vi "Tree Data Types and XML Example.vi"(0 "Show IDs (True)":bool, 1 "Tree":string(tree)) -> (12 "XML String":string)   [LabVIEW 2016, in "Tree Manager.lvclass"]
uses:
  Tree Manager.lvclass
  Data Types/String/String.lvclass/String.ctl
  Data Types/Bool/Bool.lvclass/Bool.ctl
  Data Types/Float/Float.lvclass/Float.ctl
  Data Types/Int/Integer.lvclass/Integer.ctl
  Data Types/Path/Path.lvclass/Path.ctl
  Data Types/Float/To Float Tree Data.vi
  Data Types/Bool/To Bool Tree Data.vi
  Data Types/Path/To Path Tree Data.vi
  Data Types/Int/To Integer Tree Data.vi
  Data Types/String/To String Tree Data.vi
  Data Types/Bool/Bool.lvclass
  C:/Users/plkruczp/Google Drive/MyCode/Modules/Tree/Tree Data/Tree Data.lvclass
  Data Types/Float/Float.lvclass
  Data Types/Int/Integer.lvclass
  Data Types/Path/Path.lvclass
  Data Types/String/String.lvclass
  API/List Roots.vi
  API/Set Attribute Tree Data.vi
  Tree Data/Tree Data.lvclass
  Data Types/Int/From Integer Tree Data.vi
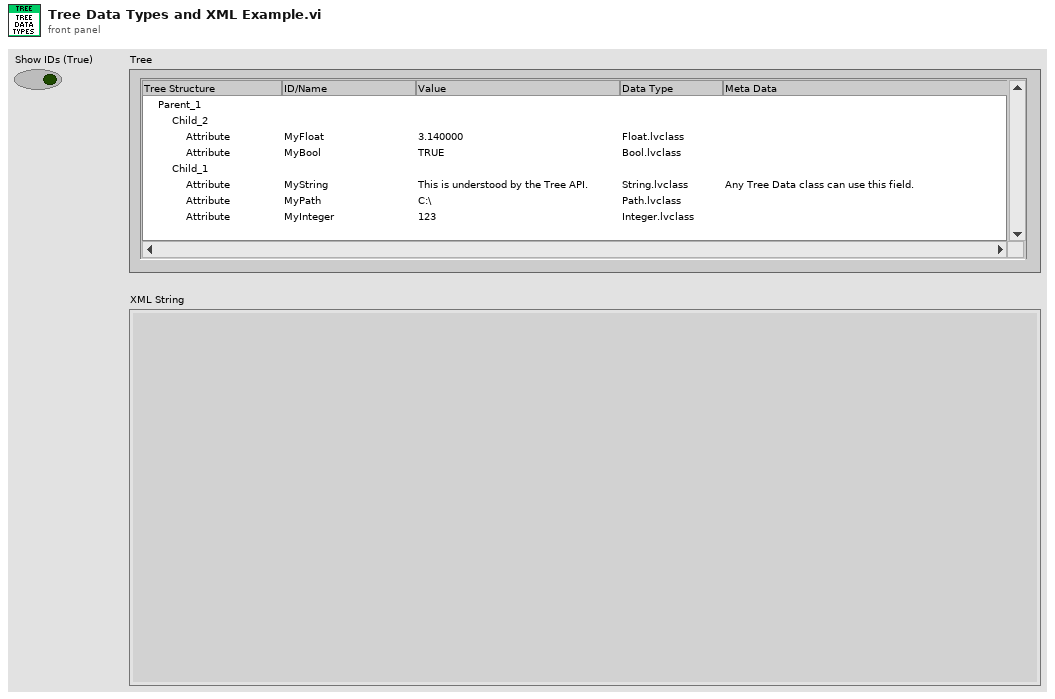
[diagram p1: front panel]
types:
  T1 = typedef "Tree Manager.lvclass/Session Handle.ctl" = refnum<data-value>
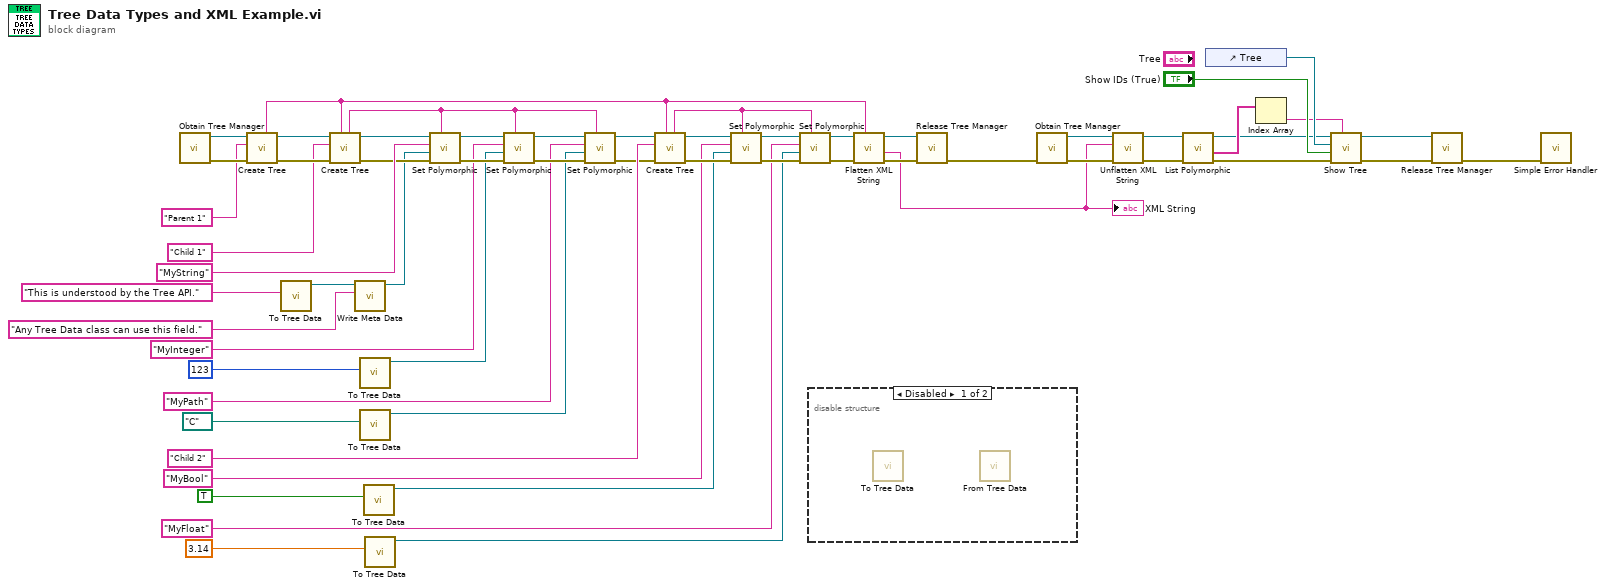
[diagram p0: block diagram]
diagram:
  n1 = call "Obtain Tree Manager.vi"() -> ("Error Out"=w57:errorcluster, "Tree Manager"=w58:T1)  [unwired: 10 in]
  n2 = call "Create Tree.vi"("Error In"=w57, "Name"="Parent 1", "Tree Manager"=w58) -> ("Error Out"=w55:errorcluster, "Tree Manager"=w56:T1, "Unique ID"=w13:string)  [unwired: 6 in]
  n3 = call-poly "To Tree Data.vi"("String"="This is understood by the Tree API.") -> ("String Tree Data"=w22:refnum<class "String.lvclass">)  [unwired: 10 in]
  n4 = call "Create Tree.vi"("Parent ID (empty)"=w13, "Error In"=w55, "Name"="Child 1", "Tree Manager"=w56) -> ("Error Out"=w45:errorcluster, "Tree Manager"=w47:T1, "Unique ID"=w21:string)  [unwired: 5 in]
  n5 = call "Write Meta Data.vi"("Meta Data"="Any Tree Data class can use this field.", "Tree Data In"=w22) -> ("Tree Data Out"=w44:refnum<class "String.lvclass">)  [unwired: 9 in]
  n6 = call-poly "To Tree Data.vi"("Integer"=i64 123) -> ("Integer Tree Data"=w24:refnum<class "Integer.lvclass">)  [unwired: 10 in]
  n7 = call-poly "To Tree Data.vi"("Path"=path "C:/") -> ("Path Tree Data"=w26:refnum<class "Path.lvclass">)  [unwired: 10 in]
  n8 = call-poly "To Tree Data.vi"("Boolean"=TRUE) -> ("Bool Tree Data"=w28:refnum<class "Bool.lvclass">)  [unwired: 10 in]
  n9 = call-poly "To Tree Data.vi"("Float"=3.14) -> ("Float Tree Data"=w30:refnum<class "Float.lvclass">)  [unwired: 10 in]
  n10 = call-poly "Set Polymorphic.vi"("Tree ID"=w21, "Error In"=w45, "Attribute Value"=w44, "Attribute Name"="MyString" ("Name"), "Tree Manager"=w47) -> ("Error Out"=w38:errorcluster, "Tree Manager"=w39:T1)  [unwired: 4 in, 1 out]
  n11 = call-poly "Set Polymorphic.vi"("Tree ID"=w21, "Error In"=w38, "Attribute Value"=w24, "Attribute Name"="MyInteger" ("Name"), "Tree Manager"=w39) -> ("Error Out"=w35:errorcluster, "Tree Manager"=w36:T1)  [unwired: 4 in, 1 out]
  n12 = call-poly "Set Polymorphic.vi"("Tree ID"=w21, "Error In"=w35, "Attribute Value"=w26, "Attribute Name"="MyPath" ("Name"), "Tree Manager"=w36) -> ("Error Out"=w33:errorcluster, "Tree Manager"=w34:T1)  [unwired: 4 in, 1 out]
  n13 = call "Create Tree.vi"("Parent ID (empty)"=w13, "Error In"=w33, "Name"="Child 2", "Tree Manager"=w34) -> ("Error Out"=w49:errorcluster, "Tree Manager"=w50:T1, "Unique ID"=w20:string)  [unwired: 5 in]
  n14 = call-poly "Set Polymorphic.vi"("Tree ID"=w20, "Error In"=w49, "Attribute Value"=w28, "Attribute Name"="MyBool" ("Name"), "Tree Manager"=w50) -> ("Error Out"=w41:errorcluster, "Tree Manager"=w42:T1)  [unwired: 4 in, 1 out]
  n15 = call-poly "Set Polymorphic.vi"("Tree ID"=w20, "Error In"=w41, "Attribute Value"=w30, "Attribute Name"="MyFloat" ("Name"), "Tree Manager"=w42) -> ("Error Out"=w14:errorcluster, "Tree Manager"=w15:T1)  [unwired: 4 in, 1 out]
  n16 = disable-structure shown="Disabled" {
    frame Disabled {
      n17 = call-poly "To Tree Data.vi"() -> ()  [unwired: 11 in, 1 out]
      n18 = call-poly "From Tree Data.vi"() -> ()  [unwired: 11 in, 1 out]
    }
    frame Enabled {
    }
  }
  n19 = call "Flatten XML String.vi"("Root ID"=w13, "Error In"=w14, "Tree Manager"=w15) -> ("Error Out"=w11:errorcluster, "XML String"=w1:string, "Tree Manager"=w12:T1)  [unwired: 6 in]
  "XML String" <- w1
  n20 = call "Release Tree Manager.vi"("Error In"=w11, "Tree Manager"=w12) -> ("Error Out"=w10:errorcluster)  [unwired: 9 in]
  n21 = call "Obtain Tree Manager.vi"("Error In"=w10) -> ("Error Out"=w8:errorcluster, "Tree Manager"=w9:T1)  [unwired: 9 in]
  n22 = call "Unflatten XML String.vi"("Error In"=w8, "XML String"=w1, "Tree Manager"=w9) -> ("Error Out"=w6:errorcluster, "Tree Manager"=w7:T1)  [unwired: 7 in]
  n23 = call-poly "List Polymorphic.vi"("Error In"=w6, "Tree Manager"=w7) -> ("Error Out"=w3:errorcluster, "Roots IDs"=w5:string[], "Tree Manager"=w4:T1)  [unwired: 6 in, 1 out]
  n24 = control-ref of="Tree"() -> (w51:refnum<vi>)
  n25 = Index Array(array=w5) -> (element=w2:string)  [unwired: 1 in]
  n26 = call "Show Tree.vi"("Root ID"=w2, "Error In"=w3, "Show IDs (True)"="Show IDs (True)", "Tree Ref"=w51, "Tree Manager"=w4) -> ("Error Out"=w18:errorcluster, "Tree Manager"=w19:T1)  [unwired: 5 in]
  n27 = call "Release Tree Manager.vi"("Error In"=w18, "Tree Manager"=w19) -> ("Error Out"=w16:errorcluster)  [unwired: 9 in]
  n28 = call <vilib>:"Simple Error Handler.vi"("error in (no error)"=w16) -> ()  [unwired: 4 in, 5 out]
